vi "ZCAN_SetRecvMerge.vi"(0 "device_handle":u32, 2 "can通道":i32, 3 "error in (no error)":errorcluster caption="错误输入（无错误）") -> (7 "device_handle(out)":u32, 8 "enable_success?":bool, 10 "error out":errorcluster caption="错误输出")   [LabVIEW 2018]
doc: "该函数用于关闭设备，关闭设备和打开设备一一对应。\n\n调用该函数，会关闭整个CAN设备（对于设备句柄），不分通道。"
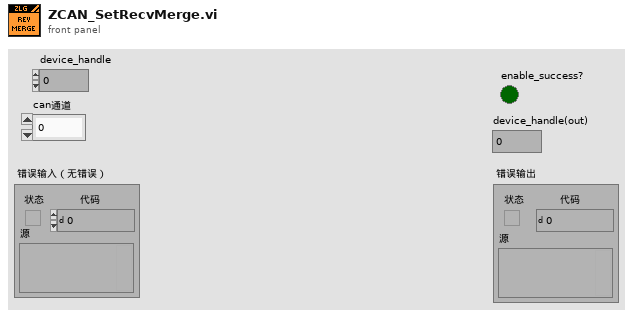
[diagram p1: front panel]
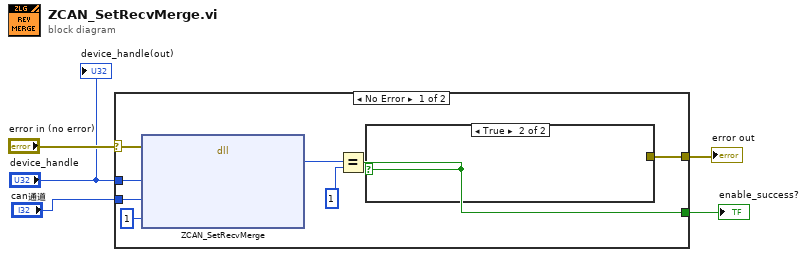
[diagram p0: block diagram]
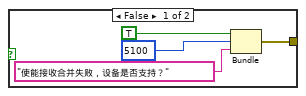
[diagram p2: hidden frame]
diagram:
  n1 = case shown="No Error" "error in (no error)" {
    selector: "error in (no error)" -> [w8 w18]
    tunnel: [w11 w18] -> w4
    tunnel: "device_handle" -> [w13 _]
    tunnel: [w9 _] -> w2
    tunnel: "can通道" -> [w7 _]
    frame No Error {
      n2 = dll-call lib="PTH2kabs CUsersadminDesktopzlgcan_demo_20220516_2018版本zlgcan_demo_USBCANFDbinzlgcan_wrap.dll" fn="ZCAN_SetRecvMerge" ("ZCAN_StartCAN")(error in=w8, "device_handle"=w13, "can通道"=w7, "使能"=1) -> ("return"=w10:u32)  [unwired: 5 in, 2 out]
      n3 = Equal?(x=w10, y=1) -> (x = y?=w9:bool)
      n4 = case shown="True" w9 {
        tunnel: [w14 _] -> w11
        frame False {
          n5 = Bundle("status"=TRUE, "code"=5100, "消息"="使能接收合并失败，设备是否支持？") -> (w14:cluster{"status":bool, "code":i32, "消息":string})  [unwired: 1 in]
        }
        frame True {
        }
      }
    }
    frame Error {
    }
  }
  "error out" <- w4
  "enable_success?" <- w2
  "device_handle(out)" <- "device_handle"
